vi "Open Gyro.vi"(8 "error in (no error)":errorcluster) -> (0 "error out":errorcluster)   [LabVIEW 2018]
uses:
  TypeDefs/typedef_enum_Refnums.ctl
  <vilib>/Rock Robotics/WPI/ThirdParty/Phoenix-LabVIEW/Pigeon IMU/CTRE_PigeonIMU_Open_CAN.vi
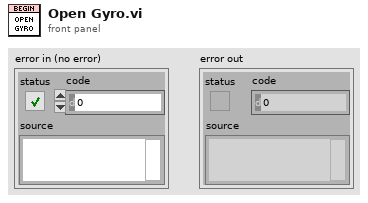
[diagram p1: front panel]
types:
  T1 = typedef "typedef_enum_Refnums.ctl" = enum16{"Ball_Encoder", "Ball_Motor", "Camera", "Linefollow_3", "Linefollow_2", "Linefollow_1", "Gyro", "Hatch_Solenoid", "Climb_Back_Solenoid", "Arm_Encoder", "Arm_Motor", "Lift_Encoder", "Drive", "Drive_Motor_R", "Drive_Motor_L", "Drive_Encoder_R", "Drive_Encoder_L", "Joy_R", "Joy_L", "Wrist_Motor", "Wrist_Encoder", "Climb Upper Limit", "Climb Lower Limit ", "Climb_Front_Motor"}
  T2 = typedef "CTRE_PigeonIMU_DeviceRef.ctl" = cluster{"DeviceStatus":errorcluster, "Device Number":u8, "Type":T3, "Device ID":u32, "Handle":u64, "UsageFrame":u32, "Library Path":path}
  T3 = typedef "CTRE_PigeonIMU_ConnectionType.ctl" = u32
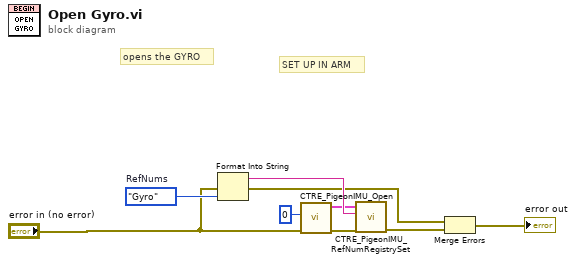
[diagram p0: block diagram]
diagram:
  w8 = typedef_enum_Refnums."Gyro"  # RefNums
  # "SET UP IN ARM"
  # "opens the GYRO"
  n1 = Format Into String(error in="error in (no error)", w8) -> (resulting string=w7:string, error out=w4:errorcluster)  [unwired: 2 in]
  n2 = call-poly <vilib>:"CTRE_PigeonIMU_Open.vi"("error in"="error in (no error)", "Device Number"=u8 0) -> ("error out"=w9:errorcluster, "PigeonIMUDevRef"=w1:T2)  [unwired: 8 in]
  n3 = call <vilib>:"CTRE_PigeonIMU_RefNumRegistrySet.vi"("error in (no error)"=w9, "refnum name"=w7, "PigeonIMUDevRef"=w1) -> ("error out"=w5:errorcluster)  [unwired: 7 in, 1 out]
  n4 = Merge Errors(w4, w5) -> (→"error out":errorcluster)
